vi "svx_Colormap Text Position.vi"(4 "Test size":i16, 5 "String":string, 11 "End":cluster{"x":i16, "y":i16}={"x"=135, "y"=0}) -> (3 "text position":cluster{"x":i16, "y":i16})   [LabVIEW 2017, in "SVX Colormap.xctl"]
uses:
  <vilib>/addons/_XControls/Colormap/SVX Colormap.xctl
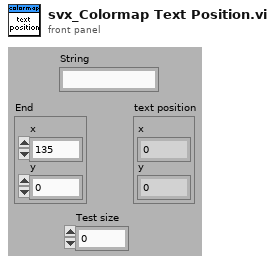
[diagram p1: front panel]
types:
  T1 = cluster{"horizontal":enum16{"left", "center", "right"}, "vertical":enum16{"top", "center", "bottom"}}
  T2 = enum16{"None", "Stacked", "Clockwise", "Counterclockwise"}
  T3 = cluster{"Font Name:":string, "Size":i16, "Strikeout?":bool, "Italic?":bool, "Underline?":bool, "Outline?":bool, "Shadow?":bool, "Bold?":bool}
  T4 = enum16{"User-specified Font", "Application Font", "System Font", "Dialog Font"}
  T5 = cluster{"left":i16, "top":i16, "right":i16, "bottom":i16}
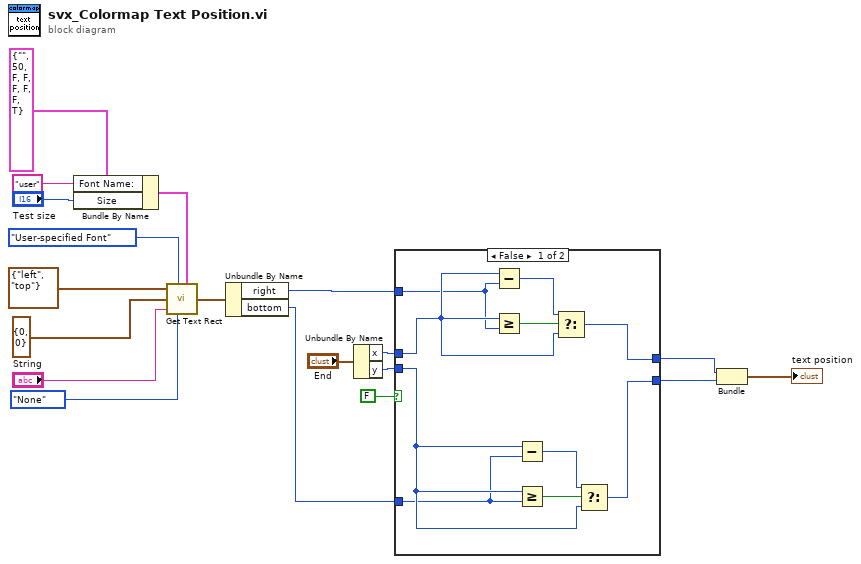
[diagram p0: block diagram]
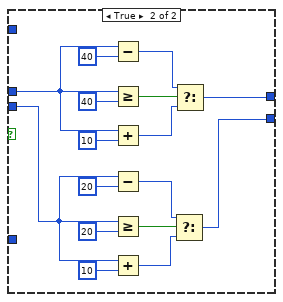
[diagram p2: hidden frame]
diagram:
  n1 = Bundle By Name(cluster=T3 {"Font Name:"="", "Size"=50, "Strikeout?"=FALSE, "Italic?"=FALSE, "Underline?"=FALSE, "Outline?"=FALSE, "Shadow?"=FALSE, "Bold?"=TRUE} ("[user-specified font]"), "Font Name:"="user", "Size"="Test size") -> (w7:T3)
  n2 = call <vilib>:"Get Text Rect.vi"("alignment(left, top)"=T1 {"horizontal"=enum."left", "vertical"=enum."top"}, "desired font(Application)"=T4."User-specified Font", "origin(0,0)"=cluster{"x":i16, "y":i16} {"x"=0, "y"=0} ("origin"), "text"="String", "text orientation"=T2."None", "[user-specified font]"=w7) -> ("rect"=w3:T5)  [unwired: 3 in]
  n3 = Unbundle By Name(w3) -> ("right"=w2:i16, "bottom"=w1:i16)
  n4 = Unbundle By Name("End") -> ("x"=w17:i16, "y"=w15:i16)
  n5 = case shown="False" FALSE {
    tunnel: w17 -> [w26 w41]
    tunnel: [w27 w38] -> w16
    tunnel: w15 -> [w22 w31]
    tunnel: [w20 w30] -> w14
    tunnel: w2 -> [w25 _]
    tunnel: w1 -> [w21 _]
    frame False {
      n6 = Subtract(x=w26, y=w25) -> (x-y=w28:i16)
      n7 = Greater Or Equal?(x=w26, y=w25) -> (x >= y?=w29:bool)
      n8 = Subtract(x=w22, y=w21) -> (x-y=w24:i16)
      n9 = Greater Or Equal?(x=w22, y=w21) -> (x >= y?=w23:bool)
      n10 = Select(t=w28, s=w29, f=w26) -> (s? t:f=w27:i16)
      n11 = Select(t=w24, s=w23, f=w22) -> (s? t:f=w20:i16)
    }
    frame True {
      n12 = Subtract(x=w41, y=i16 40) -> (x-y=w42:i16)
      n13 = Greater Or Equal?(x=w41, y=i16 40) -> (x >= y?=w44:bool)
      n14 = Add(x=w41, y=i16 10) -> (x+y=w39:i16)
      n15 = Subtract(x=w31, y=i16 20) -> (x-y=w35:i16)
      n16 = Greater Or Equal?(x=w31, y=i16 20) -> (x >= y?=w33:bool)
      n17 = Add(x=w31, y=i16 10) -> (x+y=w37:i16)
      n18 = Select(t=w35, s=w33, f=w37) -> (s? t:f=w30:i16)
      n19 = Select(t=w42, s=w44, f=w39) -> (s? t:f=w38:i16)
    }
  }
  n20 = Bundle("x"=w16, "y"=w14) -> (→"text position":cluster{"x":i16, "y":i16})  [unwired: 1 in]
